vi "Teleop.vi"(10 "Match Info":T1={"Autonomous Elapsed Seconds"=0.0, "TeleOp Elapsed Seconds"=0.0, "Disabled Elapsed Seconds"=0.0, "Visited Autonomous"=FALSE, "Visited TeleOp"=FALSE, "Visited Disabled"=FALSE, "Autonomous Settings"={"Autonomous Style"=enum."Independent", "VI Refnum"=refnum}}, 11 "Call Context":T2) -> ()   [LabVIEW 2016]
doc: "This VI is called for each TeleOp packet received from the DS where the robot is not disabled. It is often used to read from the joysticks and update I/O or to update setpoints for timed control loops. It should complete and return within 20 milliseconds or it may miss DS packets."
uses:
  <vilib>/Rock Robotics/WPI/DriverStation/WPI_DriverStationDerivedRobotMode.ctl
  <vilib>/Rock Robotics/WPI/DriverStation/WPI_DriverStationMatch Info.ctl
  <vilib>/Rock Robotics/WPI/Utilities/WPI_GetSetVariantRefNum.vi
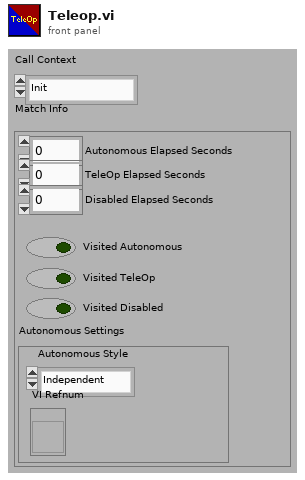
[diagram p1: front panel]
types:
  T1 = typedef "WPI_DriverStationMatch Info.ctl" = cluster{"Autonomous Elapsed Seconds":dbl, "TeleOp Elapsed Seconds":dbl, "Disabled Elapsed Seconds":dbl, "Visited Autonomous":bool, "Visited TeleOp":bool, "Visited Disabled":bool, "Autonomous Settings":cluster{"Autonomous Style":enum16{"Iterative", "Independent"}, "VI Refnum":refnum<vi>}}
  T2 = typedef "WPI_DriverStationDerivedRobotMode.ctl" = enum16{"Init", "Execute", "Stop"}
  T3 = typedef "WPI_JoystickDevRef.ctl" = cluster{"Device":T4}
  T4 = typedef "WPI_JoystickDeviceEnum.ctl" = enum16{"USB 0", "USB 1", "USB 2", "USB 3", "USB 4", "USB 5"}
  T5 = typedef "WPI_MotorControlDeviceRef.ctl" = cluster{"DeviceStatus":errorcluster, "Type":T6, "PWM":cluster{"PWM Channel":T7, "DeadBand":T8}, "CAN":cluster{"Device Number":u8, "SetOutput VI Ref":variant, "GetOutput VI Ref":variant, "Enable VI Ref":variant, "Disable VI Ref":variant, "Data":variant}, "Invert":bool}
  T6 = typedef "WPI_MotorControlType.ctl" = enum16{"PWM", "CAN"}
  T7 = typedef "FPGA_DIOPWMChannel.ctl" = enum8{"PWM 0", "PWM 1", "PWM 2", "PWM 3", "PWM 4", "PWM 5", "PWM 6", "PWM 7", "PWM 8", "PWM 9", "PWM MXP 0", "PWM MXP 1", "PWM MXP 2", "PWM MXP 3", "PWM MXP 4", "PWM MXP 5", "PWM MXP 6", "PWM MXP 7", "PWM MXP 8", "PWM MXP 9", "Invalid"}
  T8 = typedef "WPI_PWMDeadband.ctl" = cluster{"Name":string, "maxPositivePwm":i32, "minPositivePwm":i32, "centerPwm":i32, "maxNegativePwm":i32, "minNegativePwm":i32, "angularRange":u16}
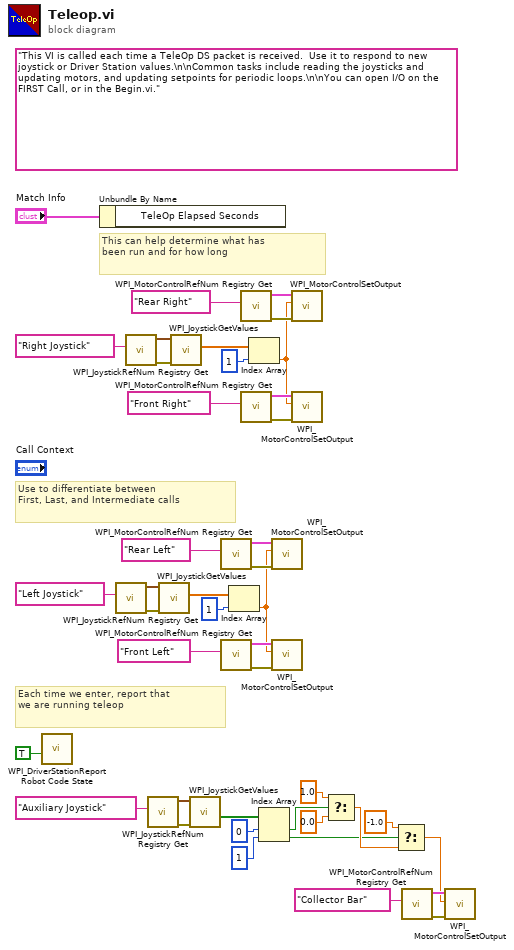
[diagram p0: block diagram]
diagram:
  (unwired) "This VI is called each time a TeleOp DS packet is received.  Use it to respond to new joystick or Driver Station values.\n\nCommon tasks include reading the joysticks and updating motors, and updating setpoints for periodic loops.\n\nYou can open I/O on the FIRST Call, or in the Begin.vi."
  # "Each time we enter, report that\nwe are running teleop"
  # "Use to differentiate between\nFirst, Last, and Intermediate calls"
  # "This can help determine what has\nbeen run and for how long"
  n1 = call <vilib>:"WPI_DriverStationReport Robot Code State.vi"("TeleOp"=TRUE ("Autonomous")) -> ()  [unwired: 10 in, 1 out]
  n2 = Unbundle By Name("Match Info") -> ()  [unwired: 1 out]
  n3 = call <vilib>:"WPI_JoystickRefNum Registry Get.vi"("refnum name"="Left Joystick") -> ("error out"=w27:errorcluster, "JoystickDevRef"=w26:T3)  [unwired: 9 in]
  n4 = call <vilib>:"WPI_JoystickRefNum Registry Get.vi"("refnum name"="Right Joystick") -> ("error out"=w39:errorcluster, "JoystickDevRef"=w38:T3)  [unwired: 9 in]
  n5 = call <vilib>:"WPI_JoystickRefNum Registry Get.vi"("refnum name"="Auxiliary Joystick") -> ("error out"=w15:errorcluster, "JoystickDevRef"=w14:T3)  [unwired: 9 in]
  n6 = call <vilib>:"WPI_JoystickGetValues.vi"("error in (no error)"=w27, "JoystickDevRef"=w26) -> ("Axes"=w25:dbl[])  [unwired: 5 in, 4 out]
  n7 = call <vilib>:"WPI_JoystickGetValues.vi"("error in (no error)"=w39, "JoystickDevRef"=w38) -> ("Axes"=w37:dbl[])  [unwired: 5 in, 4 out]
  n8 = call <vilib>:"WPI_JoystickGetValues.vi"("error in (no error)"=w15, "JoystickDevRef"=w14) -> ("Buttons"=w13:bool[])  [unwired: 5 in, 4 out]
  n9 = call <vilib>:"WPI_MotorControlRefNum Registry Get.vi"("refnum name"="Rear Left") -> ("error out"=w22:errorcluster, "MotorControlDevRef"=w21:T5)  [unwired: 9 in]
  n10 = call <vilib>:"WPI_MotorControlRefNum Registry Get.vi"("refnum name"="Front Left") -> ("error out"=w19:errorcluster, "MotorControlDevRef"=w18:T5)  [unwired: 9 in]
  n11 = Index Array(array=w25, index=1) -> (element=w17:dbl)
  n12 = call <vilib>:"WPI_MotorControlRefNum Registry Get.vi"("refnum name"="Rear Right") -> ("error out"=w34:errorcluster, "MotorControlDevRef"=w33:T5)  [unwired: 9 in]
  n13 = call <vilib>:"WPI_MotorControlRefNum Registry Get.vi"("refnum name"="Front Right") -> ("error out"=w31:errorcluster, "MotorControlDevRef"=w30:T5)  [unwired: 9 in]
  n14 = Index Array(array=w37, index=1) -> (element=w29:dbl)
  n15 = Index Array(array=w13, index #1=0 ("index"), index #2=1 ("index")) -> (element #1=w11:bool, element #2=w5:bool)
  n16 = call <vilib>:"WPI_MotorControlSetOutput.vi"("error in (no error)"=w22, "Output"=w17, "MotorControlDevRef"=w21) -> ()  [unwired: 6 in, 3 out]
  n17 = call <vilib>:"WPI_MotorControlSetOutput.vi"("error in (no error)"=w19, "Output"=w17, "MotorControlDevRef"=w18) -> ()  [unwired: 6 in, 3 out]
  n18 = call <vilib>:"WPI_MotorControlSetOutput.vi"("error in (no error)"=w34, "Output"=w29, "MotorControlDevRef"=w33) -> ()  [unwired: 6 in, 3 out]
  n19 = call <vilib>:"WPI_MotorControlSetOutput.vi"("error in (no error)"=w31, "Output"=w29, "MotorControlDevRef"=w30) -> ()  [unwired: 6 in, 3 out]
  n20 = Select(t=1.0, s=w11, f=0.0) -> (s? t:f=w8:dbl)
  n21 = Select(t=-1.0, s=w5, f=w8) -> (s? t:f=w1:dbl)
  n22 = call <vilib>:"WPI_MotorControlRefNum Registry Get.vi"("refnum name"="Collector Bar") -> ("error out"=w3:errorcluster, "MotorControlDevRef"=w2:T5)  [unwired: 9 in]
  n23 = call <vilib>:"WPI_MotorControlSetOutput.vi"("error in (no error)"=w3, "Output"=w1, "MotorControlDevRef"=w2) -> ()  [unwired: 6 in, 3 out]
